vi "Move Asset by ID.vi"(8 "error in (no error)":errorcluster, 10 "Location":string, 11 "Asset ID":string) -> (0 "error out":errorcluster)   [LabVIEW 2021]
uses:
  <vilib>/NI/Advanced HTTP Client/Header--Combo Box.ctl
  <vilib>/NI/Advanced HTTP Client/POST (Buffer).vi
  <vilib>/NI/Advanced HTTP Client/Session.lvclass
  <vilib>/Skyline/Configuration/HTTP/NI Skyline Configuration Library.lvlib
panel:
  out "url":string
  out "body":string
  out "buffer":string
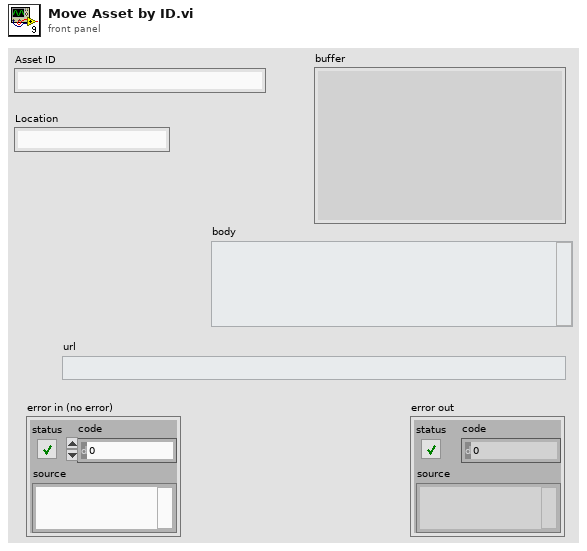
[diagram p1: front panel]
types:
  T1 = typedef "lib_NI_Advanced HTTP Client.lvlib/Session.lvclass/Header--Combo Box.ctl" = string
  T2 = typedef "NI Skyline Configuration Library.lvlib/Auto Configuration.ctl" = cluster{"id":string, "uri":string, "api key":string, "cert path":path, "owning file":path}
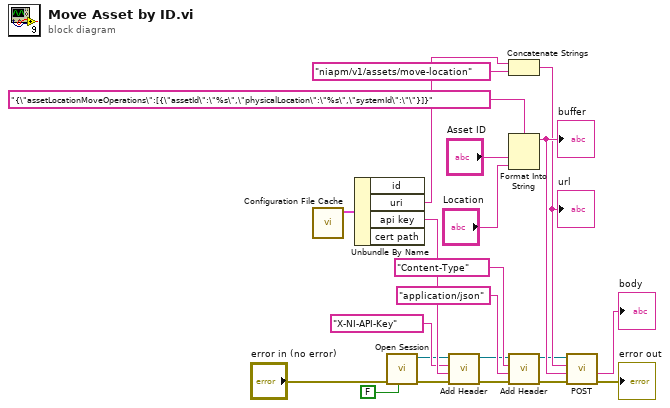
[diagram p0: block diagram]
diagram:
  n1 = call <vilib>:"Configuration File Cache.vi"() -> ("HTTP configuration"=w14:T2)  [unwired: 10 in, 1 out]
  n2 = Unbundle By Name(w14) -> ("uri"=w19:string, "api key"=w18:string)  [unwired: 2 out]
  n3 = call <vilib>:"Open Session.vi"("verify server (T)"=FALSE, "error in"="error in (no error)") -> ("error out"=w16:errorcluster, "session"=w15:refnum<class "Session.lvclass">)  [unwired: 8 in]
  n4 = call <vilib>:"Add Header.vi"("error in"=w16, "value"=w18, "header"=T1 "X-NI-API-Key", "session in"=w15) -> ("error out"=w3:errorcluster, "session out"=w4:refnum<class "Session.lvclass">)  [unwired: 6 in]
  n5 = Concatenate Strings(w19, "niapm/v1/assets/move-location" ("url")) -> (w7:string)
  "url" <- w7
  n6 = Format Into String(format string="{\"assetLocationMoveOperations\":[{\"assetId\":\"%s\",\"physicalLocation\":\"%s\",\"systemId\":\"\"}]}" ("JSON"), "Asset ID", "Location") -> (resulting string=w22:string)  [unwired: 2 in, 1 out]
  "buffer" <- w22
  n7 = call <vilib>:"Add Header.vi"("error in"=w3, "value"="application/json", "header"=T1 "Content-Type", "session in"=w4) -> ("error out"=w1:errorcluster, "session out"=w2:refnum<class "Session.lvclass">)  [unwired: 6 in]
  n8 = call-poly <vilib>:"POST.vi"("error in"=w1, "buffer"=w22, "url"=w7, "session in"=w2) -> ("error out"=→"error out":errorcluster, "body"=→"body":string)  [unwired: 3 in, 3 out]
